vi "Register Entities.vi"(8 "error in (no error)":errorcluster, 10 "Entities":refnum<class "Entity.lvclass">[](array[class]), 11 "Entity Manager in":refnum<class "Entity Manager.lvclass">) -> (0 "error out":errorcluster, 3 "Entity Manager out":refnum<class "Entity Manager.lvclass">)   [LabVIEW 2020, in "Conditu2.lvlib" / "Entity Manager.lvclass"]
uses:
  Entity Manager.lvclass
  Entity/Entity.lvclass
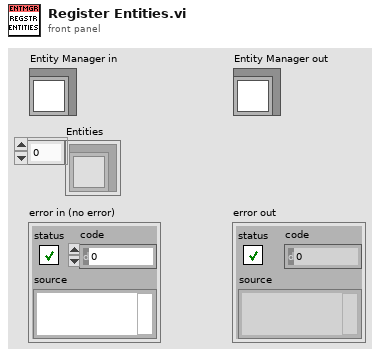
[diagram p1: front panel]
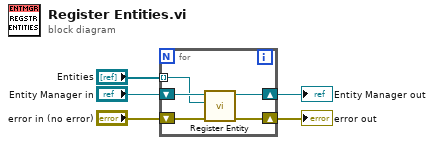
[diagram p0: block diagram]
diagram:
  n1 = for {
    tunnel: "Entities" -> [w6] mode=indexing
    shift-right: [w8] -> w2
    shift-left: "Entity Manager in" -> [w10]
    shift-right: [w7] -> w1
    shift-left: "error in (no error)" -> [w9]
    n2 = call "Register Entity.vi"("error in (no error)"=w9, "Entity"=w6, "Entity Manager in"=w10) -> ("error out"=w7:errorcluster, "Entity Manager out"=w8:refnum<class "Entity Manager.lvclass">)  [unwired: 7 in]
  }
  "error out" <- w1
  "Entity Manager out" <- w2
